vi "MeasureData.vi"(5 "Reset?":bool, 7 "Write?":bool, 8 "error in":errorcluster caption="错误输入", 9 "Measure Voltage":dbl, 10 "Measure Power":dbl, 11 "Measure Current":dbl) -> (0 "error out":errorcluster caption="错误输出", 1 "PowerAverage(..10)":dbl, 2 "CurrentAverage(..10)":dbl, 3 "VoltageAverage(..10)":dbl)   [LabVIEW 2020]
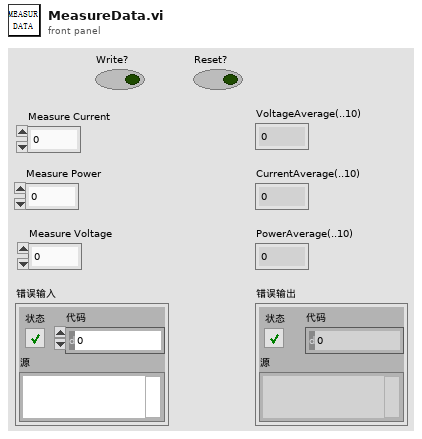
[diagram p1: front panel]
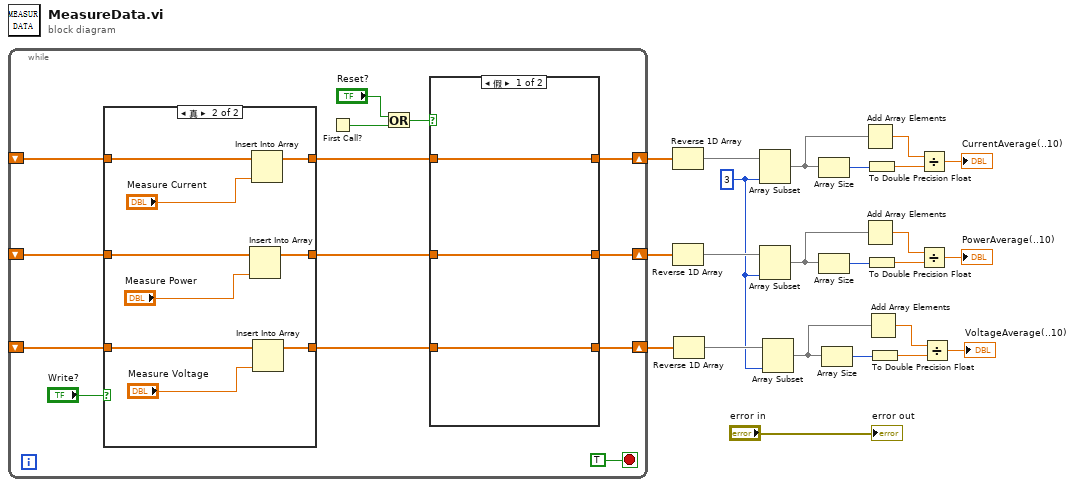
[diagram p0: block diagram]
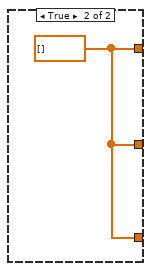
[diagram p3: hidden frame]
diagram:
  w2 = 3 ("长度")
  n1 = while {
    shift-right: [w31] -> w23
    shift-left: _ -> [w37]
    shift-right: [w30] -> w22
    shift-left: _ -> [w36]
    shift-right: [w29] -> w21
    shift-left: _ -> [w35]
    stop <- TRUE stop-if-true
    n2 = case shown="真" "Write?" {
      tunnel: w37 -> [w40 w48]
      tunnel: w36 -> [w39 w47]
      tunnel: w35 -> [w38 w44]
      tunnel: [w40 w43] -> w34
      tunnel: [w39 w42] -> w33
      tunnel: [w38 w41] -> w32
      frame False {
      }
      frame True {
        n3 = Insert Into Array(array=w47, new element="Measure Power") -> (w42:dbl[])  [unwired: 1 in]
        n4 = Insert Into Array(array=w48, new element="Measure Current") -> (w43:dbl[])  [unwired: 1 in]
        n5 = Insert Into Array(array=w44, new element="Measure Voltage") -> (w41:dbl[])  [unwired: 1 in]
      }
    }
    n6 = First Call?() -> (First Call?: T/F=w26:bool)
    n7 = Or(x="Reset?", y=w26) -> (x .or. y?=w24:bool)
    n8 = case shown="假" w24 {
      tunnel: w34 -> [w52 _]
      tunnel: w33 -> [w51 _]
      tunnel: w32 -> [w50 _]
      tunnel: [w52 w53] -> w31
      tunnel: [w51 w53] -> w30
      tunnel: [w50 w53] -> w29
      frame False {
      }
      frame True {
        w53 = dbl[] []
      }
    }
  }
  n9 = Reverse 1D Array(array=w23) -> (reversed array=w20:dbl[])
  n10 = Reverse 1D Array(array=w22) -> (reversed array=w9:dbl[])
  n11 = Reverse 1D Array(array=w21) -> (reversed array=w3:dbl[])
  n12 = Array Subset(array=w20, length=w2) -> (w19:dbl[])  [unwired: 1 in]
  n13 = Array Subset(array=w9, length=w2) -> (w10:dbl[])  [unwired: 1 in]
  n14 = Array Subset(array=w3, length=w2) -> (w8:dbl[])  [unwired: 1 in]
  n15 = Array Size(array=w19) -> (size(s)=w17:i32)
  n16 = Array Size(array=w10) -> (size(s)=w12:i32)
  n17 = Array Size(array=w8) -> (size(s)=w6:i32)
  n18 = Add Array Elements(numeric array=w19) -> (sum=w18:dbl)
  n19 = Add Array Elements(numeric array=w10) -> (sum=w11:dbl)
  n20 = To Double Precision Float(number=w17) -> (double precision float=w16:dbl)
  n21 = To Double Precision Float(number=w12) -> (double precision float=w13:dbl)
  n22 = Add Array Elements(numeric array=w8) -> (sum=w7:dbl)
  n23 = To Double Precision Float(number=w6) -> (double precision float=w5:dbl)
  n24 = Divide(x=w18, y=w16) -> (x/y=→"CurrentAverage(..10)":dbl)
  n25 = Divide(x=w11, y=w13) -> (x/y=→"PowerAverage(..10)":dbl)
  n26 = Divide(x=w7, y=w5) -> (x/y=→"VoltageAverage(..10)":dbl)
  "error out" <- "error in"
